vi "ACDC_Config_9234.vi"(8 "error in (no error)":errorcluster, 9 "Input Config Array":T1[](array[typedef])=[0, 0, 0, 0, 0, 0, 0, 0, 0, 0, 0, 0, 0, 0, 0, 0, 0, 0, 0, 0, 0, 0, 0, 0, 0, 0, 0, 0, 0, 0, 0, 0] items=["AC Coupled", "DC Coupled", "IEPE AC Coupled"], 10 "Data Rate [S/s]":u32) -> (0 "error out":errorcluster)   [LabVIEW 2017, in "BOP_VibAPI_4.lvlib"]
uses:
  <vilib>/addons/InsightCM/Devices/Shared/Cms/Fpga/Acquisition/source/subVIs/VibAPI_4/BOP_VibAPI_4.lvlib
  <vilib>/LabVIEW Targets/FPGA/cRIO/shared/nicrio_ModuleControls/nicrio_cRIO-9232_ConfigModeRing.ctl
  <vilib>/rvi/eio/common/nirviEmuTemplatePropertySet_errors.vi
  <vilib>/eio/EIOPropertyNode/EIOPropertyNode.xnode
  <vilib>/LabVIEW Targets/FPGA/cRIO/shared/nicrio_ModuleControls/nicrio_cRIO-9234_DataRatesRing2.ctl
  <vilib>/LabVIEW Targets/FPGA/cRIO/shared/nicrio_ModuleControls/nicrio_cRIO-9234_ConfigModeRing.ctl
  <vilib>/rvi/eio/common/nirviEmuTemplatePropertyGet_errors.vi
  <vilib>/rvi/eio/common/nirviEmuTemplatePropertyGet_noerrors.vi
  <vilib>/rvi/eio/common/nirviEmuTemplatePropertySet_noerrors.vi
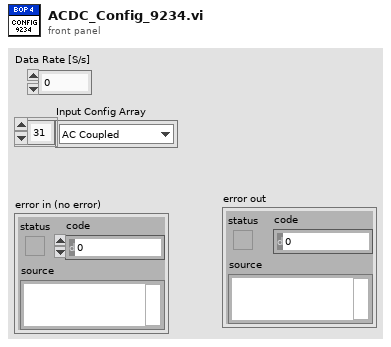
[diagram p1: front panel]
types:
  T1 = typedef "nicrio_cRIO-9232_ConfigModeRing.ctl" = u8
  T2 = typedef "nicrio_cRIO-9234_DataRatesRing2.ctl" = u8
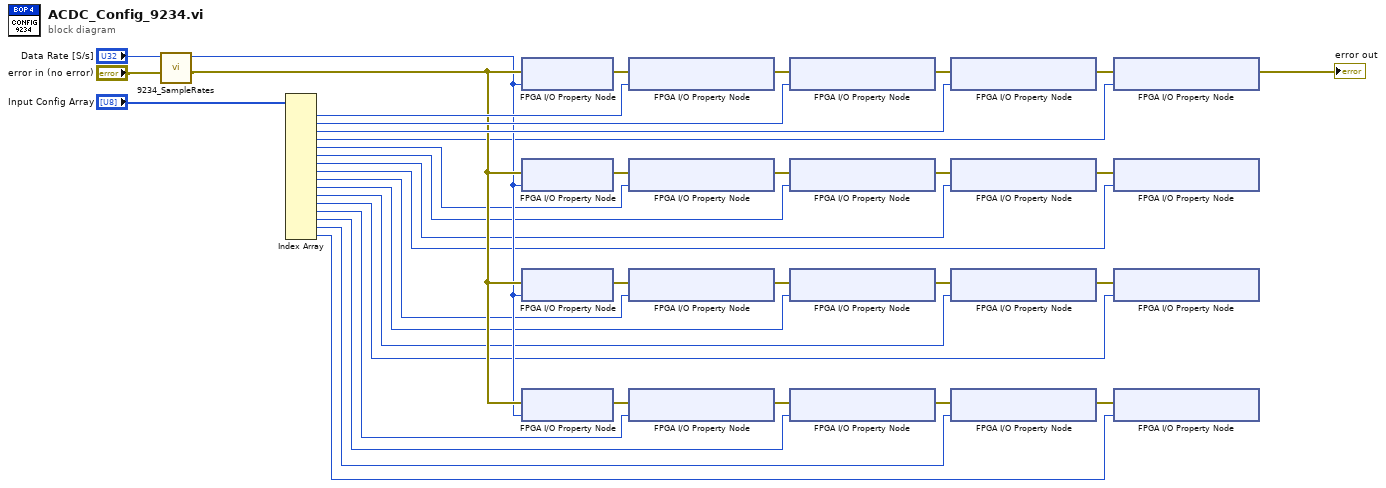
[diagram p0: block diagram]
diagram:
  n1 = call <vilib>:"9234_SampleRates.vi"("error in (no error)"="error in (no error)", "Data Rate [S/s]"="Data Rate [S/s]") -> ("error out"=w20:errorcluster, "Data Rate"=w19:T2)  [unwired: 8 in]
  n2 = Index Array(array="Input Config Array") -> (element #1=w30:T1, element #2=w29:T1, element #3=w28:T1, element #4=w5:T1, element #5=w7:T1, element #6=w8:T1, element #7=w9:T1, element #8=w6:T1, element #9=w11:T1, element #10=w12:T1, element #11=w13:T1, element #12=w10:T1, element #13=w15:T1, element #14=w16:T1, element #15=w17:T1, element #16=w14:T1)  [unwired: 16 in]
  n3 = xnode "FPGA I/O Property Node"("error in"=w20, "Data Rate"=w19) -> ("error out"=w32:errorcluster)  [unwired: 1 in, 1 out]
  n4 = xnode "FPGA I/O Property Node"("error in"=w20, "Data Rate"=w19) -> ("error out"=w31:errorcluster)  [unwired: 1 in, 1 out]
  n5 = xnode "FPGA I/O Property Node"("error in"=w20, "Data Rate"=w19) -> ("error out"=w24:errorcluster)  [unwired: 1 in, 1 out]
  n6 = xnode "FPGA I/O Property Node"("error in"=w20, "Data Rate"=w19) -> ("error out"=w23:errorcluster)  [unwired: 1 in, 1 out]
  n7 = xnode "FPGA I/O Property Node"("error in"=w32, "Input Configuration"=w30) -> ("error out"=w33:errorcluster)  [unwired: 1 in, 1 out]
  n8 = xnode "FPGA I/O Property Node"("error in"=w31, "Input Configuration"=w7) -> ("error out"=w35:errorcluster)  [unwired: 1 in, 1 out]
  n9 = xnode "FPGA I/O Property Node"("error in"=w24, "Input Configuration"=w11) -> ("error out"=w25:errorcluster)  [unwired: 1 in, 1 out]
  n10 = xnode "FPGA I/O Property Node"("error in"=w23, "Input Configuration"=w15) -> ("error out"=w22:errorcluster)  [unwired: 1 in, 1 out]
  n11 = xnode "FPGA I/O Property Node"("error in"=w33, "Input Configuration"=w29) -> ("error out"=w34:errorcluster)  [unwired: 1 in, 1 out]
  n12 = xnode "FPGA I/O Property Node"("error in"=w35, "Input Configuration"=w8) -> ("error out"=w36:errorcluster)  [unwired: 1 in, 1 out]
  n13 = xnode "FPGA I/O Property Node"("error in"=w25, "Input Configuration"=w12) -> ("error out"=w26:errorcluster)  [unwired: 1 in, 1 out]
  n14 = xnode "FPGA I/O Property Node"("error in"=w22, "Input Configuration"=w16) -> ("error out"=w21:errorcluster)  [unwired: 1 in, 1 out]
  n15 = xnode "FPGA I/O Property Node"("error in"=w34, "Input Configuration"=w28) -> ("error out"=w18:errorcluster)  [unwired: 1 in, 1 out]
  n16 = xnode "FPGA I/O Property Node"("error in"=w36, "Input Configuration"=w9) -> ("error out"=w4:errorcluster)  [unwired: 1 in, 1 out]
  n17 = xnode "FPGA I/O Property Node"("error in"=w26, "Input Configuration"=w13) -> ("error out"=w3:errorcluster)  [unwired: 1 in, 1 out]
  n18 = xnode "FPGA I/O Property Node"("error in"=w21, "Input Configuration"=w17) -> ("error out"=w2:errorcluster)  [unwired: 1 in, 1 out]
  n19 = xnode "FPGA I/O Property Node"("error in"=w18, "Input Configuration"=w5) -> ("error out"=→"error out":errorcluster)  [unwired: 1 in, 1 out]
  n20 = xnode "FPGA I/O Property Node"("error in"=w4, "Input Configuration"=w6) -> ()  [unwired: 1 in, 2 out]
  n21 = xnode "FPGA I/O Property Node"("error in"=w3, "Input Configuration"=w10) -> ()  [unwired: 1 in, 2 out]
  n22 = xnode "FPGA I/O Property Node"("error in"=w2, "Input Configuration"=w14) -> ()  [unwired: 1 in, 2 out]
